vi "Get Owning Project.vi"(8 "error in (no error)":errorcluster, 11 "VI in":refnum<vi>) -> (0 "error out":errorcluster, 1 "owning project ref":refnum<vi>, 2 "owning project name":string, 3 "VI out":refnum<vi>)   [LabVIEW 2017]
doc: "Returns <b>VI in</b> owner project name and reference."
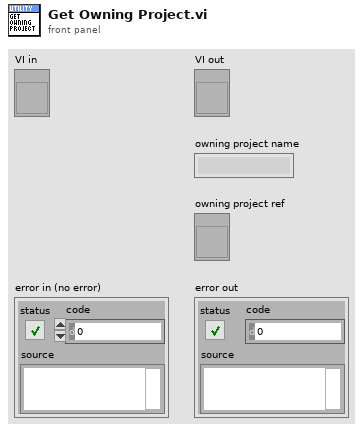
[diagram p1: front panel]
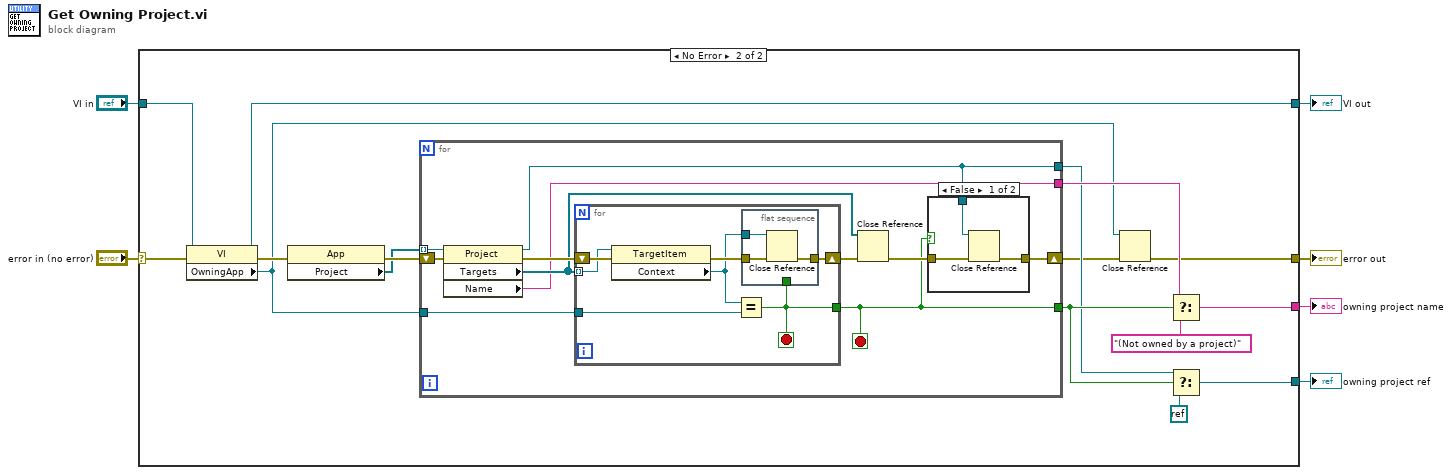
[diagram p0: block diagram]
diagram:
  n1 = case shown="No Error" "error in (no error)" {
    selector: "error in (no error)" -> [w8 w9]
    tunnel: [_ w20] -> w6
    tunnel: "VI in" -> [w7 w17]
    tunnel: [_ w13] -> w4
    tunnel: [w7 w11] -> w3
    tunnel: [w8 w10] -> w1
    frame Error {
    }
    frame No Error {
      n2 = property class="VI"(reference=w17, error in=w9) -> (reference out=w11:refnum<vi>, error out=w23:errorcluster, "OwningApp"=w18:refnum<vi>)
      n3 = property class="App"(error in=w23) -> (error out=w24:errorcluster, "Project"=w19:refnum<vi>[])  [unwired: 1 in, 1 out]
      n4 = for {
        tunnel: w19 -> [w34] mode=indexing
        shift-right: [w26] -> w12
        shift-left: w24 -> [w33]
        tunnel: w18 -> [w29]
        tunnel: [w27] -> w16
        tunnel: [w28] -> w22
        tunnel: [w25] -> w15
        stop <- w27 stop-if-true
        n5 = property class="Project"(reference=w34, error in=w33) -> (reference out=w25:refnum<vi>, error out=w32:errorcluster, "Targets"=w30:refnum<vi>[], "Name"=w28:string)
        n6 = for {
          tunnel: w30 -> [w45] mode=indexing
          shift-right: [w42] -> w31
          shift-left: w32 -> [w46]
          tunnel: w29 -> [w44]
          tunnel: [w41] -> w27
          stop <- w41 stop-if-true
          n7 = property class="TargetItem"(reference=w45, error in=w46) -> (error out=w43:errorcluster, "Context"=w40:refnum<vi>)  [unwired: 1 out]
          n8 = Equal?(x=w40, y=w44) -> (x = y?=w41:bool)
          n9 = flat-sequence {
            tunnel: w43 -> [w49]
            tunnel: [w48] -> w42
            tunnel: w41 -> [_]
            tunnel: w40 -> [w47]
            frame #0 {
              n10 = Close Reference(reference=w47, error in (no error)=w49) -> (error out=w48:errorcluster)
            }
          }
        }
        n11 = Close Reference(reference=w30, error in (no error)=w31) -> (error out=w35:errorcluster)
        n12 = case shown="False" w27 {
          tunnel: w35 -> [w38 w39]
          tunnel: [w37 w39] -> w26
          tunnel: w25 -> [w36 _]
          frame False {
            n13 = Close Reference(reference=w36, error in (no error)=w38) -> (error out=w37:errorcluster)
          }
          frame True {
          }
        }
      }
      n14 = Close Reference(reference=w18, error in (no error)=w12) -> (error out=w10:errorcluster)
      n15 = Select(t=w22, s=w16, f="(Not owned by a project)") -> (s? t:f=w20:string)
      n16 = Select(t=w15, s=w16, f=refnum<k0> refnum) -> (s? t:f=w13:refnum<vi>)
    }
  }
  "owning project name" <- w6
  "VI out" <- w3
  "owning project ref" <- w4
  "error out" <- w1
